vi "KE622x -- 2182 -A Get Auto Range State.vi"(0 "622x Resource In":refnum<visa-resource-name>, 1 "Check For SCPI Errors? (T)":bool=TRUE, 11 "error in (no error)":errorcluster) -> (4 "622x Resource Out (dupl)":refnum<visa-resource-name>, 8 "Auto Range Enabled?":bool, 15 "error out":errorcluster)   [LabVIEW 2013, in "Keithly user program.lvlib"]
uses:
  Keithly user program.lvlib
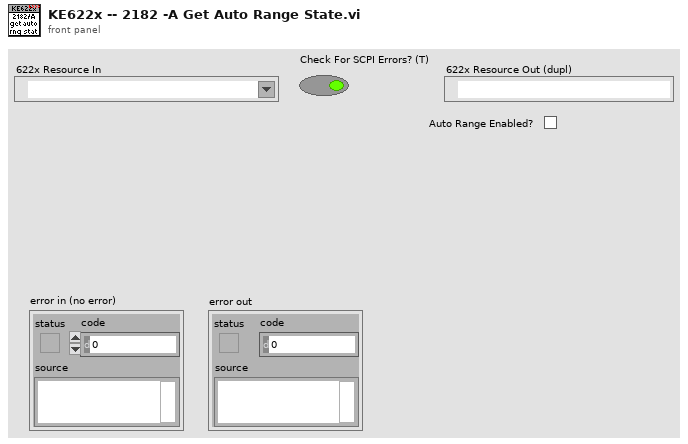
[diagram p1: front panel]
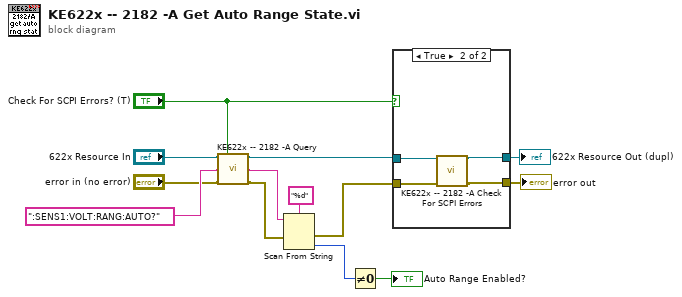
[diagram p0: block diagram]
diagram:
  n1 = call "KE622x -- 2182 -A Query.vi"("622x Resource In"="622x Resource In", "Check For SCPI Errors? (T)"="Check For SCPI Errors? (T)", "2182-A Write String"=":SENS1:VOLT:RANG:AUTO?", "error in (no error)"="error in (no error)") -> ("622x Resource Out (dupl)"=w6:refnum<visa-resource-name>, "2182-A Reponse String"=w1:string, "error out"=w2:errorcluster)  [unwired: 9 in]
  n2 = Scan From String(format string="%d", input string=w1, error in=w2) -> (error out=w12:errorcluster, output 1=w9:i32)  [unwired: 2 in, 2 out]
  n3 = Not Equal To 0?(x=w9) -> (x != 0?=→"Auto Range Enabled?":bool)
  n4 = case shown="True" "Check For SCPI Errors? (T)" {
    tunnel: w6 -> [w15 w19]
    tunnel: w12 -> [w14 w17]
    tunnel: [w15 w18] -> w11
    tunnel: [w14 w16] -> w10
    frame False {
    }
    frame True {
      n5 = call "KE622x -- 2182 -A Check For SCPI Errors.vi"("VISA Resource In"=w19, "error in (no error)"=w17) -> ("VISA Resource Out (dupl)"=w18:refnum<visa-resource-name>, "error out"=w16:errorcluster)  [unwired: 10 in, 2 out]
    }
  }
  "622x Resource Out (dupl)" <- w11
  "error out" <- w10
